vi "HTTP.Set Header.vi"(8 "error in (no error)":errorcluster, 9 "Value":string, 10 "Header Name":T1, 11 "Connection.WS in":refnum<class "Connection.WS.lvclass">) -> (0 "error out":errorcluster, 3 "Connection.WS out":refnum<class "Connection.WS.lvclass">)   [LabVIEW 2013, in "Connection.WS_GOSPL.lvlib" / "Connection.WS.lvclass"]
uses:
  Connection.WS.lvclass
  Header Fields -- combo.ctl
  Connection.WS.lvclass/Connection.WS.ctl
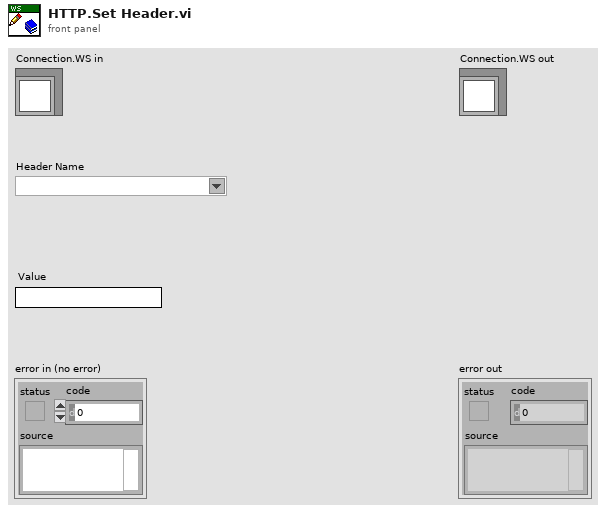
[diagram p1: front panel]
types:
  T1 = typedef "Connection.WS_GOSPL.lvlib/Connection.WS.lvclass/Header Fields -- combo.ctl" = string
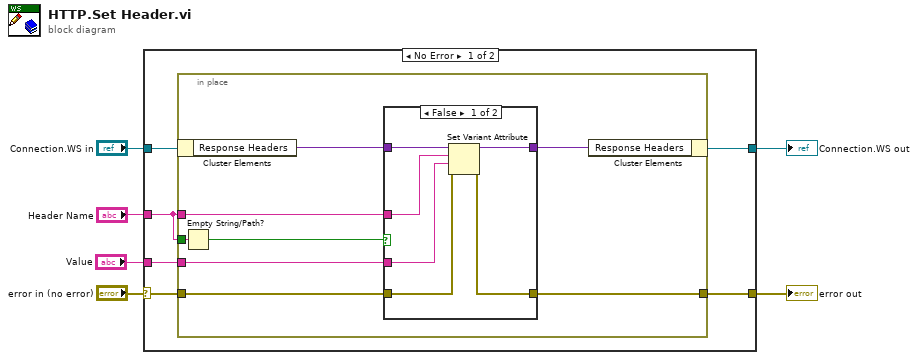
[diagram p0: block diagram]
diagram:
  n1 = case shown="No Error" "error in (no error)" {
    selector: "error in (no error)" -> [w12 w30]
    tunnel: [w11 w30] -> w5
    tunnel: [w7 w29] -> w3
    tunnel: "Connection.WS in" -> [w8 w29]
    tunnel: "Header Name" -> [w10 _]
    tunnel: "Value" -> [w13 _]
    frame No Error {
      n2 = Empty String/Path?(string/path=w10) -> (empty?=w9:bool)
      n3 = in-place {
        in-place-border: w13 -> [w20]
        in-place-border: w12 -> [w19]
        in-place-border: [w18] -> w11
        in-place-border: w10 -> [w17]
        in-place-border: w9 -> [w16]
        n4 = in-place-cluster #1(w8) -> ("Response Headers"=w15:variant)
        n5 = case shown="False" w16 {
          tunnel: w15 -> [w26 w27]
          tunnel: w20 -> [w21 _]
          tunnel: w19 -> [w25 w28]
          tunnel: [w24 w28] -> w18
          tunnel: w17 -> [w23 _]
          tunnel: [w22 w27] -> w14
          frame False {
            n6 = Set Variant Attribute(Variant=w26, name=w23, value=w21, error in=w25) -> (Variant out=w22:variant, error out=w24:errorcluster)  [unwired: 1 out]
          }
          frame True {
          }
        }
        n7 = in-place-cluster #1("Response Headers"=w14) -> (w7:refnum<class "Connection.WS.lvclass">)
      }
    }
    frame Error {
    }
  }
  "error out" <- w5
  "Connection.WS out" <- w3
